vi "Write Output_Enable.vi"(8 "error in":errorcluster, 10 "Output_Enable":bool, 11 "Acopian in":refnum<class "Acopian.lvclass">) -> (0 "error out":errorcluster, 3 "Acopian out":refnum<class "Acopian.lvclass">)   [LabVIEW 2019, in "Acopian.lvlib" / "Acopian.lvclass"]
uses:
  Library/Acopian.lvclass
  Library/Acopian.lvclass/Acopian.ctl
  builds/Instruments/PowerSupply.lvlibp/Library/PowerSupply.lvclass
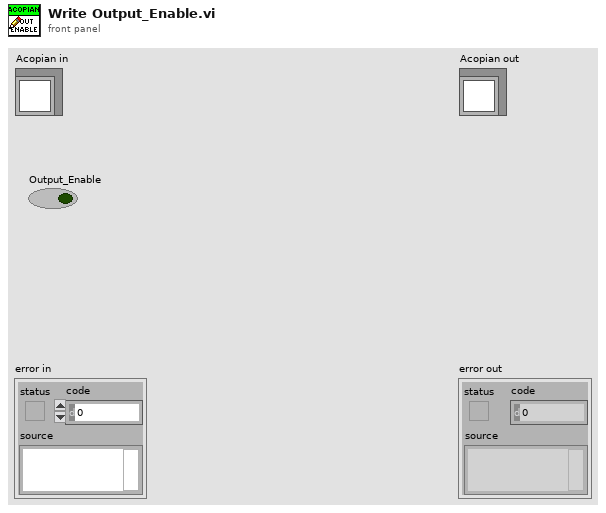
[diagram p1: front panel]
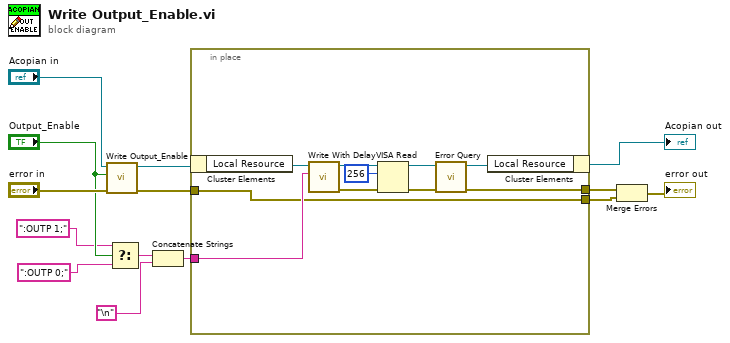
[diagram p0: block diagram]
diagram:
  n1 = call-parent "Write Output_Enable.vi"("error in"="error in", "Output_Enable"="Output_Enable", "PowerSupply in"="Acopian in") -> ("error out"=w10:errorcluster, "PowerSupply out"=w12:refnum<class "Acopian.lvclass">)  [unwired: 7 in]
  n2 = Select(t=":OUTP 1;" ("Enable/Disable Output"), s="Output_Enable", f=":OUTP 0;" ("Enable/Disable Output")) -> (s? t:f=w5:string)
  n3 = Concatenate Strings(w5, "\n") -> (w3:string)
  n4 = in-place {
    in-place-border: w10 -> [w15]
    in-place-border: w3 -> [w18]
    in-place-border: [w17] -> w6
    in-place-border: [w15] -> w1
    n5 = in-place-cluster #1(w12) -> ("Local Resource"=w22:refnum<visa-resource-name>)
    n6 = call "Write With Delay.vi"("write buffer"=w18, "VISA resource name"=w22) -> ("error out"=w19:errorcluster, "VISA resource name out"=w23:refnum<visa-resource-name>)  [unwired: 8 in]
    n7 = VISA Read(VISA resource name=w23, byte count=u32 256, error in (no error)=w19) -> (VISA resource name out=w24:refnum<visa-resource-name>, error out=w20:errorcluster)  [unwired: 2 out]
    n8 = call "Error Query.vi"("error in"=w20, "VISA resource in"=w24) -> ("error out"=w17:errorcluster, "VISA resource out"=w21:refnum<visa-resource-name>)  [unwired: 6 in, 2 out]
    n9 = in-place-cluster #1("Local Resource"=w21) -> (→"Acopian out":refnum<class "Acopian.lvclass">)
  }
  n10 = Merge Errors(w6, w1) -> (→"error out":errorcluster)
